vi "SGLToU64.vi"(5 "Number":sgl) -> (1 "Unsigned 64-bit integer":u64, 2 "Overflow?":bool, 3 "Exact conversion?":bool)   [LabVIEW 2017, in "GPOverflow.lvlib"]
doc: "Converts <B>Number</B> to U64 keeping track of numeric overflow and exactness of conversion.\n\n<B>Exact conversion?</B> will be True only if a conversion back into the original data type of <B>Number</B> will yield the exact same number, i.e. no precision was lost during the conversion.\n\n<B>Overflow?</B> will be True if positive or negative overflow occurred. The numeric output will saturate in case of overflow.\n\nThis VI is inlined.\n\nSteen Schmidt\nGPower\n9/3 2013"
uses:
  GPOverflow.lvlib
  Comparison/GPComparison.lvlib
  Comparison/Library/IsInt/IsIntSGL.vi
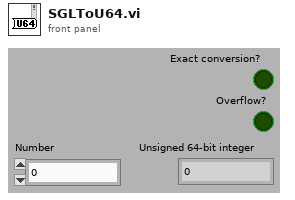
[diagram p1: front panel]
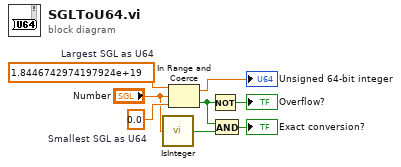
[diagram p0: block diagram]
diagram:
  w1 = sgl 1.8446743e+19  # Largest SGL as U64
  w8 = sgl 0.0  # Smallest SGL as U64
  n1 = call-poly "IsInteger.vi"("x"="Number") -> ("Integer?"=w3:bool)  [unwired: 4 in]
  n2 = In Range and Coerce(upper limit=w1, x="Number", lower limit=w8) -> (coerced(x)=→"Unsigned 64-bit integer":sgl, In Range?=w4:bool)
  n3 = Not(x=w4) -> (.not. x?=→"Overflow?":bool)
  n4 = And(x=w4, y=w3) -> (x .and. y?=→"Exact conversion?":bool)
